vi "Pairwise_distances_chunked.vi"(8 "error in":errorcluster caption="entrée d'erreur", 9 "Y":string[][](array[string]), 10 "X":string[][](array[string]), 11 "pairwise_distances_chunked":T2={"reduce_func"="None", "metric "="euclidean", "n_jobs"="None", "working_memory"="None"}) -> (0 "error out":errorcluster caption="sortie d'erreur", 3 "Data":T1)   [LabVIEW 2020]
doc: "Generate a distance matrix chunk by chunk with optional reduction\n\nIn cases where not all of a pairwise distance matrix needs to be stored at once, this is used to calculate pairwise distances in working_memory-sized chunks. If reduce_func is given, it is run on each chunk and its return values are concatenated into lists, arrays or sparse matrices.\n\nParameters :\n\n- X : array [n_samples_a, n_samples_a] if metric == “precomputed”, or,\n[n_samples_a, n_features] otherwise Array of pairwise distances between samples, or a feature array.\n\n- Y : array [n_samples_b, n_features], optional\nAn optional second feature array. Only allowed if metric != “precomputed”.\n\n- reduce_func : callable, optional\nThe function which is applied on each chunk of the distance matrix, reducing it to needed values. reduce_func(D_chunk, start) is called repeatedly, where D_chunk is a contiguous vertical slice of the pairwise distance matrix, starting at row start. It should return one of: None; an array, a list, or a sparse matrix of length D_chunk.shape[0]; or a tuple of such objects. Returning None is useful for in-place operations, rather than reductions.\n\nIf None, pairwise_distances_chunked returns a generator of vertical chunks of the distance matrix.\n\n- metric : string, or callable\nThe metric to use when calculating distance between instances in a feature array. If metric is a string, it must be one of the options allowed by scipy.spatial.distance.pdist for its metric parameter, or a metric listed in pairwise.PAIRWISE_DISTANCE_FUNCTIONS. If metric is “precomputed”, X is assumed to be a distance matrix. Alternatively, if metric is a callable function, it is called on each pair of instances (rows) and the resulting value recorded. The callable should take two arrays from X as input and return a value indicating the distance between them.\n\n- n_job : sint or None, optional (default=None)\nThe number of jobs to use for the computation. This works by breaking down the pairwise matrix into n_jobs even slices and computing them in parallel.\n\nNone means 1 unless in a joblib.parallel_backend context. -1 means using all processors. See Glossary for more details.\n\n- working_memory : int, optional\nThe sought maximum memory for temporary distance matrix chunks. When None (default), the value of sklearn.get_config()['working_memory'] is used.\n\nReturns :\n\n- D_chunk : array or sparse matrix\nA contiguous slice of distance matrix, optionally processed by reduce_func."
uses:
  Pairwise_distances_chunked.lvclass
panel:
  out "Pairwise_distances_chunked.lvclass":refnum<class "Pairwise_distances_chunked.lvclass">
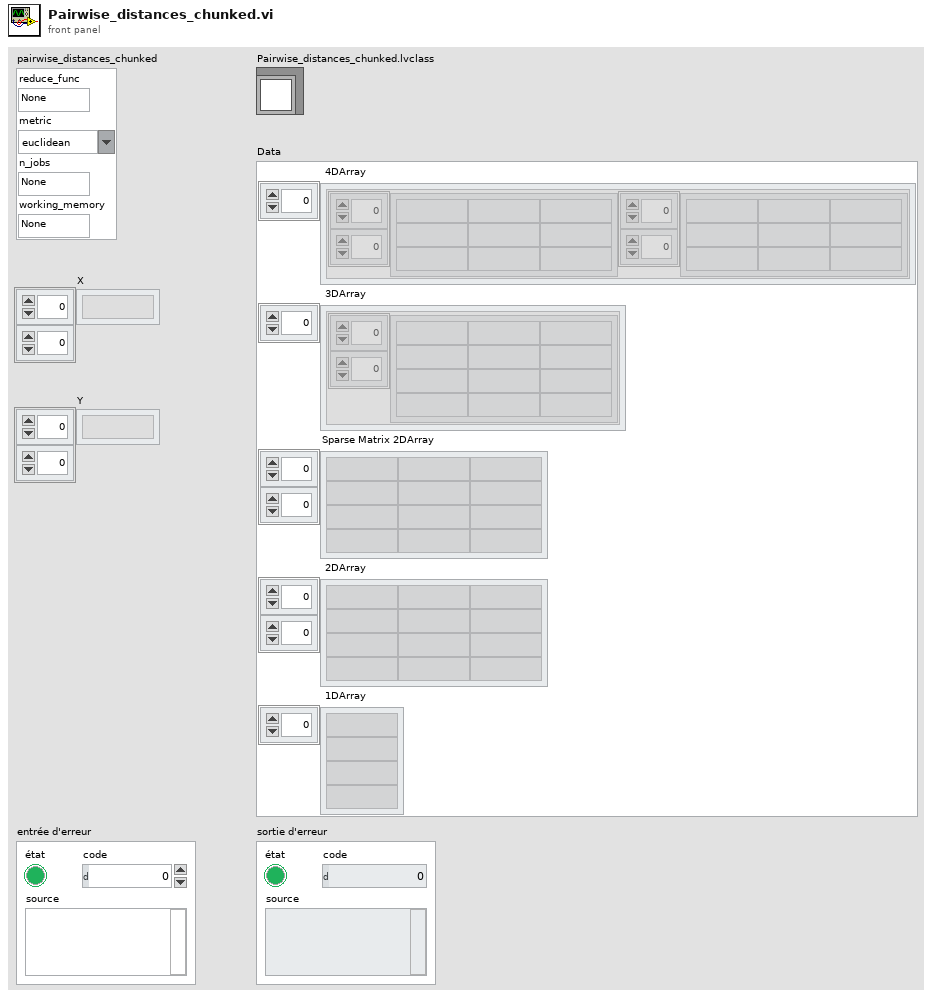
[diagram p1: front panel]
types:
  T1 = cluster{" 4DArray":cluster{"1":string[][], "2":string[][]}[], " 3DArray":cluster{"Tableau":string[][]}[], "Sparse Matrix 2DArray":string[][], " 2DArray":string[][], " 1DArray":string[]}
  T2 = cluster{"reduce_func":string, "metric ":string, "n_jobs":string, "working_memory":string}
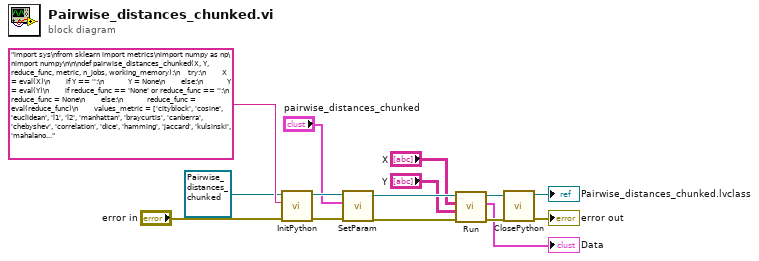
[diagram p0: block diagram]
diagram:
  n1 = call-dynamic "InitPython.vi"("error in (no error)"="error in", "Python Instruction"="import sys\nfrom sklearn import metrics\nimport numpy as np\nimport numpy\n\n\ndef pairwise_distances_chunked(X, Y, reduce_func, metric, n_jobs, working_memory):\n    try:\n        X = eval(X)\n        if Y == '':\n            Y = None\n        else:\n            Y = eval(Y)\n        if reduce_func == 'None' or reduce_func == '':\n            reduce_func = None\n        else:\n            reduce_func = eval(reduce_func)\n        values_metric = ['cityblock', 'cosine', 'euclidean', 'l1', 'l2', 'manhattan', 'braycurtis', 'canberra', 'chebyshev', 'correlation', 'dice', 'hamming', 'jaccard', 'kulsinski', 'mahalanobis', 'minkowski', 'rogerstanimoto', 'russellrao', 'seuclidean', 'sokalmichener', 'sokalsneath', 'sqeuclidean', 'yule' ]\n        if metric not in values_metric:\n            metric = eval(metric)\n        if n_jobs == 'None' or n_jobs == '':\n            n_jobs = None\n        else:\n            n_jobs = eval(n_jobs)\n        if working_memory == 'None' or working_memory == '':\n            working_memory = None\n        else:\n            working_memory = eval(working_memory)\n        pairwise_distances_chunked = metrics.pairwise_distances_chunked(X, Y, reduce_func, metric, n_jobs, working_memory)\n        pairwise_distances_chunked = next(pairwise_distances_chunked)\n        dtype = type(pairwise_distances_chunked)\n        if dtype == numpy.ndarray:\n            D_chunk = pairwise_distances_chunked.tolist()\n            return str(D_chunk)\n        else:\n            Mat = pairwise_distances_chunked.tocoo()\n            return str(list(zip(Mat.row, Mat.col, Mat.data)))\n    except:\n        erreur = sys.exc_info()\n        typerr = u\"%s\" % (erreur[0])\n        typerr = typerr[typerr.find(\"'\")+1:typerr.rfind(\"'\")]\n        msgerr = u\"%s\" % (erreur[1])\n        message = str('/!\\\\ {0} : {1}'. format(typerr,msgerr))\n        return message", "Scikit-learn en entrée"=refnum<class "Pairwise_distances_chunked.lvclass"> refnum ("Pairwise_distances_chunked.lvclass")) -> ("error out"=w6:errorcluster, "Scikit-learn en sortie"=w12:refnum<class "Pairwise_distances_chunked.lvclass">)  [unwired: 7 in]
  n2 = call-dynamic "SetParam.vi"("error in (no error)"=w6, "pairwise_distances_chunked"="pairwise_distances_chunked", "Pairwise_distances_chunked.lvclass"=w12) -> ("error out"=w10:errorcluster, "Pairwise_distances_chunked.lvclass"=w9:refnum<class "Pairwise_distances_chunked.lvclass">)  [unwired: 7 in]
  n3 = call-dynamic "Run.vi"("error in (no error)"=w10, "Y"="Y", "X"="X", "Pairwise_distances_chunked.lvclass"=w9) -> ("error out"=w7:errorcluster, "Data"=→"Data":T1, "Pairwise_distances_chunked.lvclass"=w8:refnum<class "Pairwise_distances_chunked.lvclass">)  [unwired: 5 in]
  n4 = call-dynamic "ClosePython.vi"("error in (no error)"=w7, "Scikit-learn en entrée"=w8) -> ("error out"=→"error out":errorcluster, "Scikit-learn en sortie"=→"Pairwise_distances_chunked.lvclass":refnum<class "Pairwise_distances_chunked.lvclass">)  [unwired: 8 in]
